vi "myCommOpen.vi"(8 "错误输入（无错误）":errorcluster, 10 "地址":u16, 11 "VISA引用句柄输入":refnum<visa-resource-name>) -> (0 "错误输出":errorcluster, 3 "Modbus Master输出":refnum<class "Modbus Master.lvclass">)   [LabVIEW 2024]
uses:
  <vilib>/NI/Modbus Library/API/Master/Modbus Master.lvclass
  <vilib>/NI/Modbus Library/API/Wrapper/Create Serial Master.vi
  <vilib>/NI/Modbus Library/API/Wrapper/API Main.lvlib
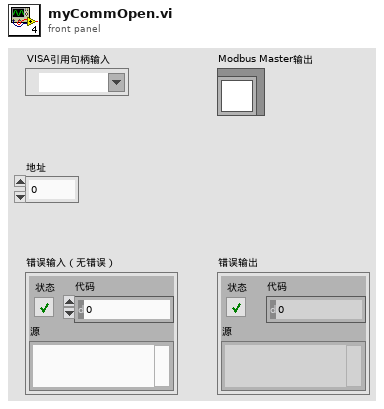
[diagram p1: front panel]
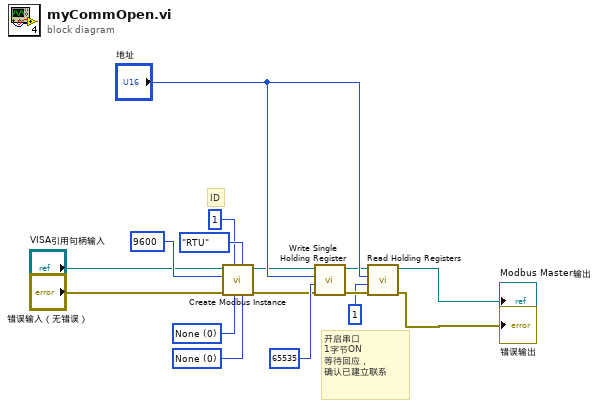
[diagram p0: block diagram]
diagram:
  w6 = u16 0 items=["None", "XON/XOFF", "RTS/CTS", "XON/XOFF & RTS/CTS", "DTR/DSR", "XON/XOFF & DTR/DSR"] ("flow control (none)")
  w5 = u16 0 items=["None", "Odd", "Even", "Mark", "Space"] ("parity (even)")
  # "开启串口\n1字节ON\n等待回应，\n确认已建立联系"
  # "ID"
  n1 = call-poly <vilib>:"Create Modbus Instance.vi"("flow control (none)"=w6, "serial type"=enum16{"RTU", "ASCII"}."RTU", "parity (even)"=w5, "unit ID"=u8 1, "error in"="错误输入（无错误）", "baud rate"=u32 9600, "VISA resource name"="VISA引用句柄输入") -> ("error out"=w11:errorcluster, "serial master instance"=w8:refnum<class "Modbus Master.lvclass">)  [unwired: 3 in]
  n2 = call-dynamic "Write Single Holding Register.vi"("error in"=w11, "register to write"=u16 65535, "address"="地址", "Modbus master in"=w8) -> ("error out"=w10:errorcluster, "Modbus master out"=w9:refnum<class "Modbus Master.lvclass">)  [unwired: 6 in]
  n3 = call-dynamic "Read Holding Registers.vi"("error in"=w10, "number of inputs"=u16 1, "starting address"="地址", "Modbus master in"=w9) -> ("error out"=→"错误输出":errorcluster, "Modbus master out"=→"Modbus Master输出":refnum<class "Modbus Master.lvclass">)  [unwired: 5 in, 1 out]
